vi "EF_createFileName.vi"(8 "FeatureExtractionParams":T2={"FeatureExtractionMethod"=enum."Amplitude Variance", "Parameter #1"=0.5, "Parameter #2"=15.0} {"Parameter #2" min=0.0 max=256.0 step=0.1; "Parameter #1" min=0.0 max=256.0 step=0.1}, 11 "Preprocessing params":T5) -> (3 "FeaturesFile Name":string)   [LabVIEW 2016, in "Feature Extraction.lvlib"]
uses:
  Feature Extraction.lvlib
  EF_SpatialFilter.ctl
  EF_FrequencyFilter.ctl
  EF_FeatureExtractionMethods.ctl
panel:
  # "This VI is a part of BCI Design library, http://www.ru-bci.org \nCopyright © 2020, Sotnikov Peter, All rights reserved. License: GNU GPLv3"
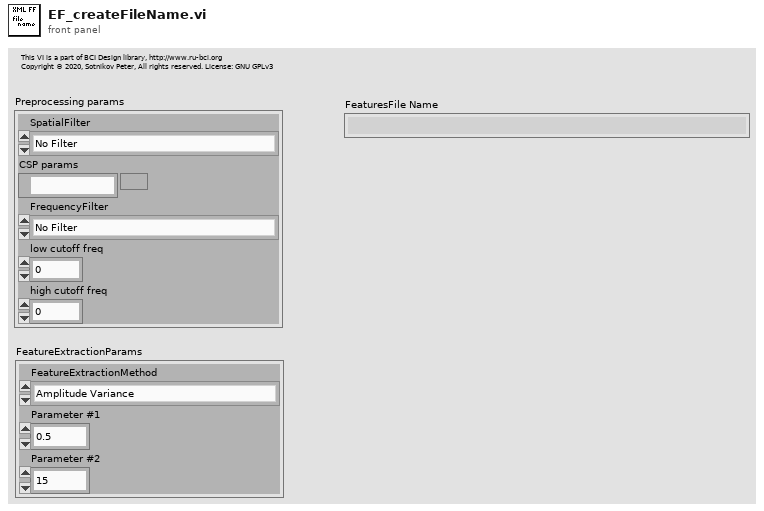
[diagram p1: front panel]
types:
  T1 = typedef "Feature Extraction.lvlib/EF_FeatureExtractionMethods.ctl" = enum16{"Amplitude Variance", "Amplitude Entropy", "EEG Spectrum (FourierTransform)", "EEG Spectrum (WaveletTransform)", "Spectral Power of EEG Rhythms (FourierTransform)", "Spectral Power of EEG Rhythms (WaveletTransform)", "Wavelet Scalogram", "Signal Downsampling", "Vector Autoregressive Model", "EEG Bicoherence"}
  T2 = cluster{"FeatureExtractionMethod":T1, "Parameter #1":dbl, "Parameter #2":dbl}
  T3 = typedef "Feature Extraction.lvlib/EF_SpatialFilter.ctl" = enum16{"No Filter", "Common Average Reference", "Common Spatial Pattern Filter", "Removal of EOG Artifacts"}
  T4 = typedef "Feature Extraction.lvlib/EF_FrequencyFilter.ctl" = enum16{"No Filter", "Kaiser Filter"}
  T5 = cluster{"SpatialFilter":T3, "CSP params":path, "FrequencyFilter":T4, "low cutoff freq":dbl, "high cutoff freq":dbl}
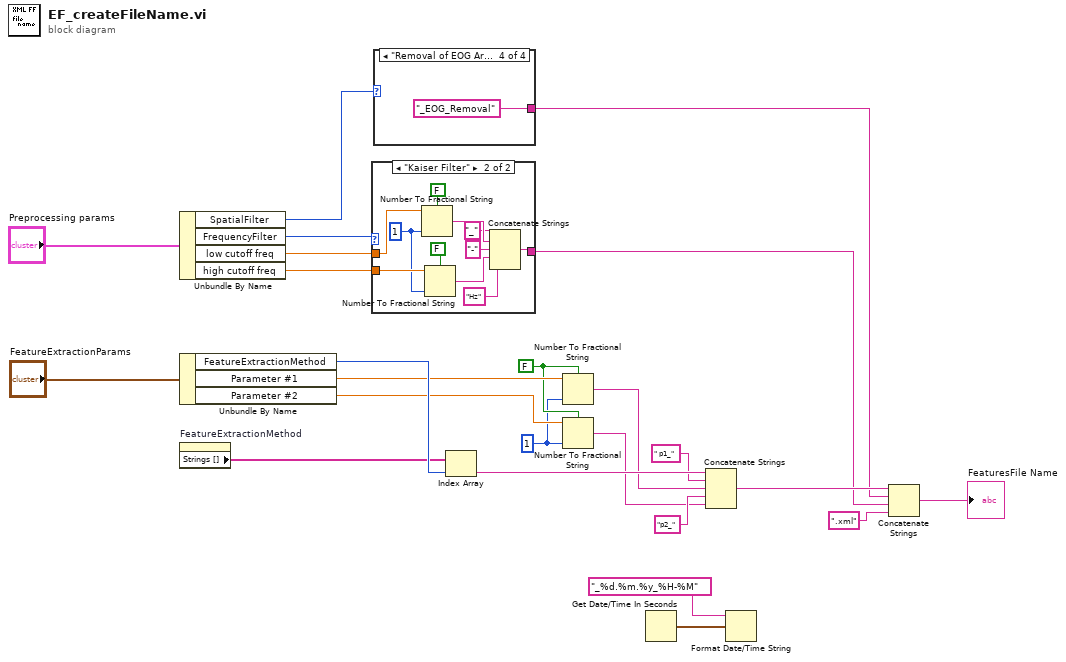
[diagram p0: block diagram]
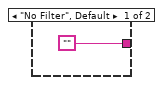
[diagram p2: hidden frame]
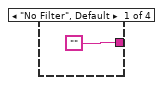
[diagram p3: hidden frame]
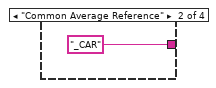
[diagram p4: hidden frame]
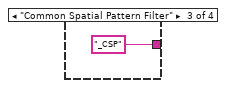
[diagram p5: hidden frame]
diagram:
  w6 = i16 1 ("precision (6)")
  w7 = FALSE ("use system decimal point (T)")
  n1 = Unbundle By Name("Preprocessing params") -> ("SpatialFilter"=w19:T3, "FrequencyFilter"=w20:T4, "low cutoff freq"=w12:dbl, "high cutoff freq"=w11:dbl)
  n2 = Unbundle By Name("FeatureExtractionParams") -> ("FeatureExtractionMethod"=w22:T1, "Parameter #1"=w9:dbl, "Parameter #2"=w8:dbl)
  n3 = property on="FeatureExtractionMethod" class="Enum (strict)"() -> ("Strings []"=w10:string[])  [unwired: 2 in, 2 out]
  n4 = case shown="\"Kaiser Filter\"" w20 {
    tunnel: ["" w31] -> w16
    tunnel: w12 -> [_ w36]
    tunnel: w11 -> [_ w34]
    frame "No Filter", Default {
    }
    frame "Kaiser Filter" {
      w33 = i16 1 ("precision (6)")
      n5 = Number To Fractional String(use system decimal point (T)=FALSE, number=w36, precision (6)=w33) -> (F-format string=w30:string)  [unwired: 1 in]
      n6 = Number To Fractional String(use system decimal point (T)=FALSE, number=w34, precision (6)=w33) -> (F-format string=w29:string)  [unwired: 1 in]
      n7 = Concatenate Strings("_" ("string"), w30, "-" ("string"), w29, "Hz" ("string")) -> (w31:string)
    }
  }
  n8 = case shown="\"Removal of EOG Artifacts\"" w19 {
    tunnel: ["" "_CAR" ("string") "_CSP" ("string") "_EOG_Removal" ("string")] -> w17
    frame "No Filter", Default {
    }
    frame "Common Average Reference" {
    }
    frame "Common Spatial Pattern Filter" {
    }
    frame "Removal of EOG Artifacts" {
    }
  }
  n9 = Index Array(array=w10, index=w22) -> (element=w21:string)
  n10 = Number To Fractional String(use system decimal point (T)=w7, number=w9, precision (6)=w6) -> (F-format string=w4:string)  [unwired: 1 in]
  n11 = Number To Fractional String(use system decimal point (T)=w7, number=w8, precision (6)=w6) -> (F-format string=w2:string)  [unwired: 1 in]
  n12 = Get Date/Time In Seconds() -> (seconds since 1Jan1904=w15:timestamp)
  n13 = Concatenate Strings(w21, " p1_" ("string"), w4, "p2_" ("string"), w2) -> (w18:string)
  n14 = Format Date/Time String(time format string (%c)="_%d.%m.%y_%H-%M", seconds (now)=w15) -> ()  [unwired: 1 in, 1 out]
  n15 = Concatenate Strings(w18, w17, w16, ".xml" ("string")) -> (→"FeaturesFile Name":string)
